vi "Exercise2Part2BTS.vi"() -> ()   [LabVIEW 2014]
panel:
  in  "stop":bool
  out "B":dbl
  out "A":dbl
  out "A+B":dbl
  # "+"
  # "="
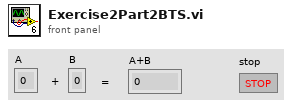
[diagram p1: front panel]
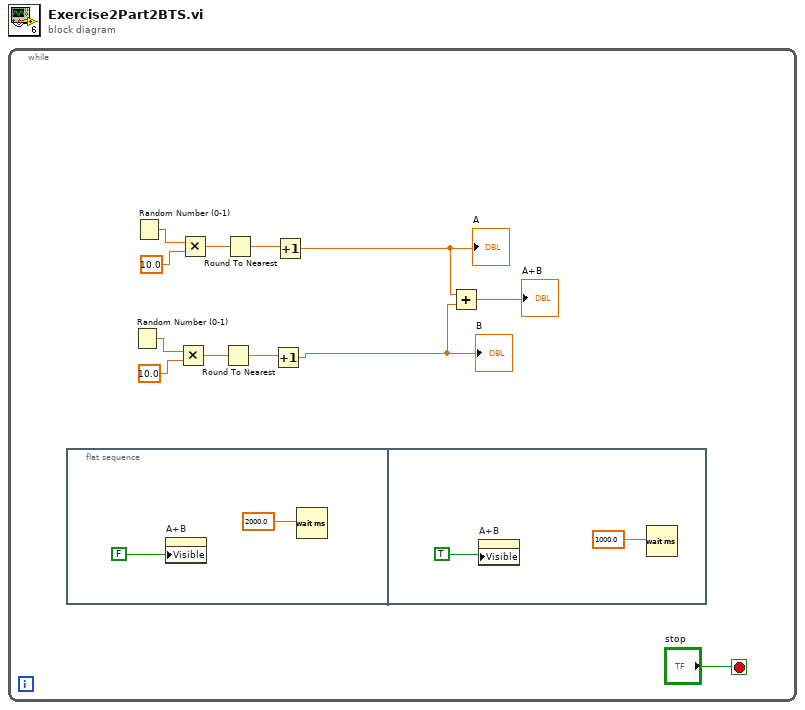
[diagram p0: block diagram]
diagram:
  n1 = while {
    stop <- "stop" stop-if-true
    n2 = flat-sequence {
      frame #0 {
        n3 = property on="A+B" class="DigNum (strict)"("Visible"=FALSE) -> ()  [unwired: 2 in, 2 out]
        n4 = Wait (ms)(milliseconds to wait=2000.0) -> ()  [unwired: 1 out]
      }
      frame #1 {
        n5 = property on="A+B" class="DigNum (strict)"("Visible"=TRUE) -> ()  [unwired: 2 in, 2 out]
        n6 = Wait (ms)(milliseconds to wait=1000.0) -> ()  [unwired: 1 out]
      }
    }
    n7 = Random Number (0-1)() -> (number: 0 to 1=w7:dbl)
    n8 = Random Number (0-1)() -> (number: 0 to 1=w11:dbl)
    n9 = Multiply(x=w7, y=10.0) -> (x*y=w5:dbl)
    n10 = Multiply(x=w11, y=10.0) -> (x*y=w9:dbl)
    n11 = Round To Nearest(number=w5) -> (nearest integer value=w4:dbl)
    n12 = Round To Nearest(number=w9) -> (nearest integer value=w8:dbl)
    n13 = Increment(x=w4) -> (x+1=w2:dbl)
    "B" <- w2
    n14 = Increment(x=w8) -> (x+1=w3:dbl)
    "A" <- w3
    n15 = Add(x=w3, y=w2) -> (x+y=→"A+B":dbl)
  }
